vi "Update_Data_Dummy.vi"(8 "error in (no error)":errorcluster, 10 "Event Data":variant, 11 "DNL_LabVIEW Object in":refnum<class>) -> (0 "error out":errorcluster, 3 "DNL_LabVIEW Object out":refnum<class>)   [LabVIEW 2017]
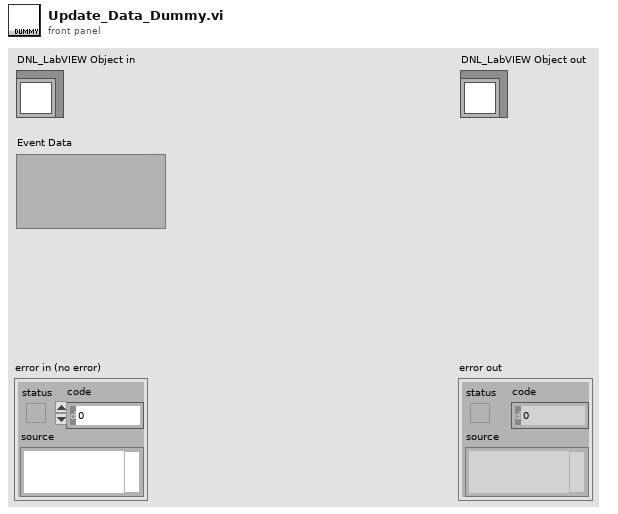
[diagram p1: front panel]
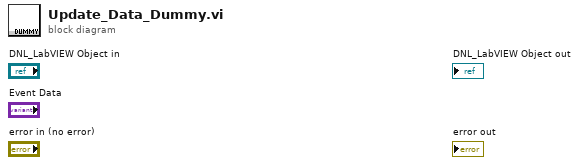
[diagram p0: block diagram]
diagram:
